vi "Component.vi"(6 "Teller":refnum<class "Teller.lvclass">, 7 "Actor in":refnum<class "Actor.lvclass">, 9 "Error":errorcluster, 10 "Actor":refnum<class "Actor.lvclass">) -> (0 "Error out":errorcluster, 5 "Actor out":refnum<class "Actor.lvclass">)   [LabVIEW 2025, in "jettl.lvlib" / "Terminate Msg.lvlib"]
uses:
  Terminate Msg.lvlib
  Actor/Actor/Actor.lvclass
  Teller/Teller/Teller.lvclass
  Terminate Msg/Terminate Msg.lvclass
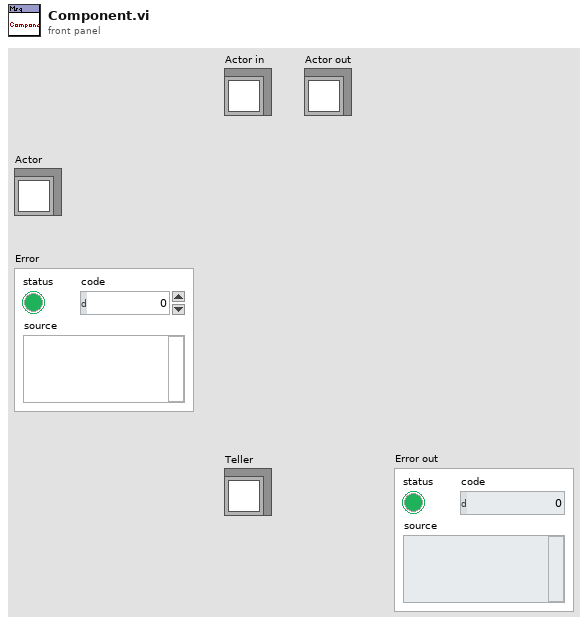
[diagram p1: front panel]
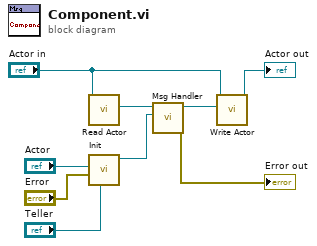
[diagram p0: block diagram]
diagram:
  n1 = call-dynamic "Read Actor.vi"("Actor in"="Actor in") -> ("Actor"=w2:refnum<class "Actor.lvclass">)  [unwired: 10 in]
  n2 = call "Init.vi"("Teller"="Teller", "Error"="Error", "Actor"="Actor") -> ("Terminate Msg out"=w8:refnum<class "Terminate Msg.lvclass">)  [unwired: 8 in]
  n3 = call-dynamic "Msg Handler.vi"("Msg"=w8, "Actor in"=w2) -> ("Error out"=→"Error out":errorcluster, "Actor out"=w1:refnum<class "Actor.lvclass">)  [unwired: 8 in]
  n4 = call-dynamic "Write Actor.vi"("Actor"=w1, "Actor in"="Actor in") -> ("Actor out"=→"Actor out":refnum<class "Actor.lvclass">)  [unwired: 9 in]
